vi "Check Valid.vi"(11 "IAction.lvclass":refnum<class "IAction.lvclass">) -> (3 "Valid?":bool)   [LabVIEW 2019, in "IAction.lvclass"]
uses:
  IAction.lvclass
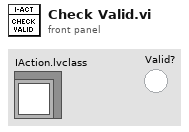
[diagram p1: front panel]
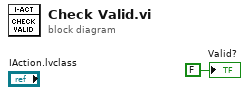
[diagram p0: block diagram]
diagram:
  "Valid?" <- FALSE ("Valid?")
